vi "checkStatus.vi"(8 "error in (no error)":errorcluster, 10 "stop":bool, 11 "Camera in":refnum<class "Camera.lvclass">) -> (0 "error out":errorcluster, 2 "stopped?":bool, 3 "Camera out":refnum<class "Camera.lvclass">)   [LabVIEW 2009, in "Hardware.lvlib" / "Channels.lvlib" / "Camera.lvclass"]
uses:
  Camera.lvclass
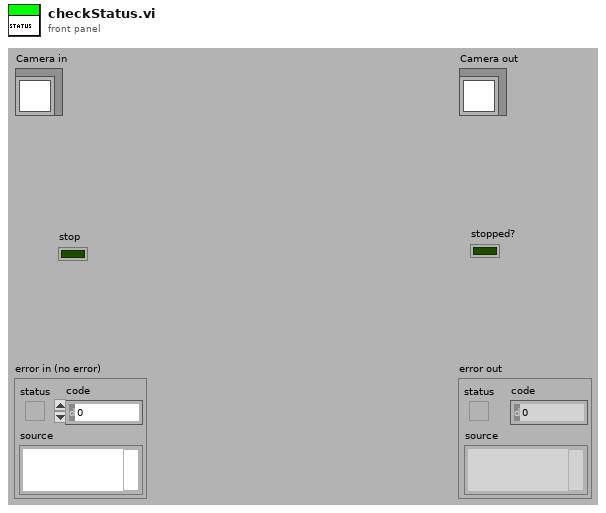
[diagram p1: front panel]
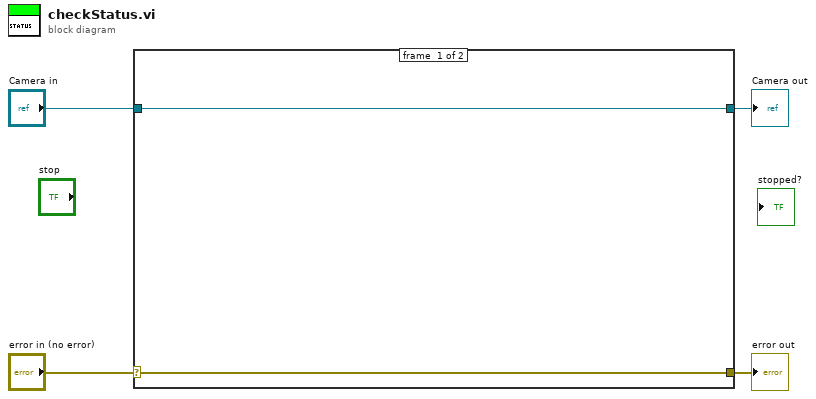
[diagram p0: block diagram]
diagram:
  n1 = case shown="No Error" "error in (no error)" {
    selector: "error in (no error)" -> [w5 w8]
    tunnel: [w5 w8] -> w3
    tunnel: [w6 w7] -> w1
    tunnel: "Camera in" -> [w6 w7]
    frame #0 {
    }
    frame #1 {
    }
  }
  "error out" <- w3
  "Camera out" <- w1
